vi "通过程序动态调整控件尺寸.vi"() -> ()   [LabVIEW 2010]
doc: "本VI是为《我和LabVIEW》一书编写的示例。\n关于本书的介绍请参考网页：\nhttp://ruanqizhen.spaces.live.com/blog/cns!5852D4F797C53FB6!4310.entry"
uses:
  C:/Program Files/National Instruments/LabVIEW 2010/resource/importtools/Common/Event/NISAST Event.lvclass
  <vilib>/Utility/miscctls.llb/LVPointTypeDef.ctl
panel:
  out "波形图":dbl[](graph)
  in  "停止":bool
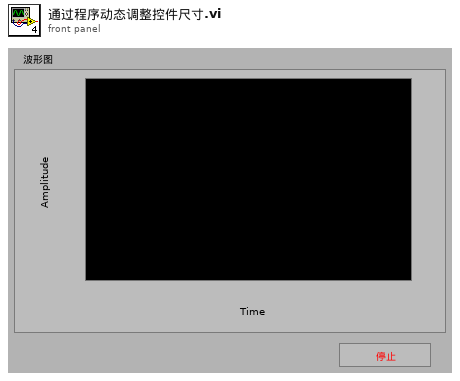
[diagram p1: front panel]
types:
  T1 = typedef "LVPointTypeDef.ctl" = cluster{"Horizontal":i16, "Vertical":i16}
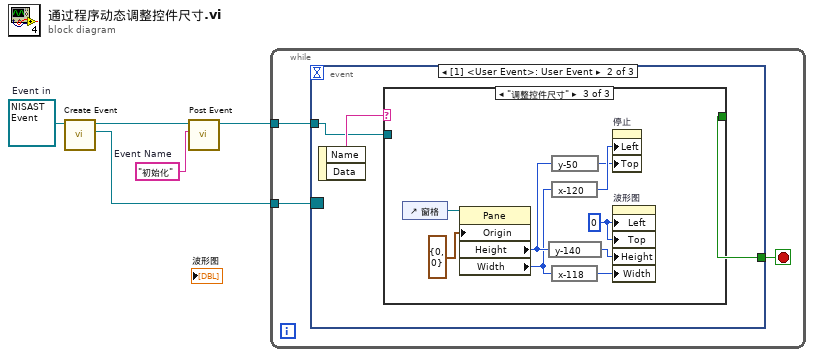
[diagram p0: block diagram]
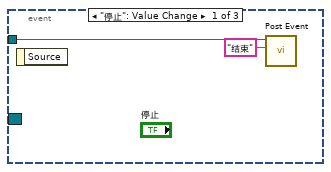
[diagram p2: hidden frame]
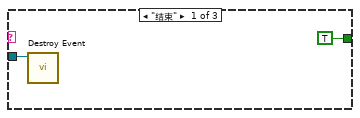
[diagram p3: hidden frame]
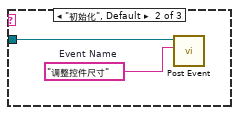
[diagram p4: hidden frame]
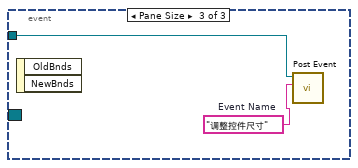
[diagram p5: hidden frame]
diagram:
  w1 = "初始化"  # Event Name
  w4 = refnum<class "NISAST Event.lvclass"> refnum  # Event in
  n1 = call-dynamic "Create Event.vi"("Event in"=w4) -> ("Event Registration Refnum"=w5:refnum<event-registration>, "Event out"=w3:refnum<class "NISAST Event.lvclass">)  [unwired: 1 in, 8 out]
  n2 = call-dynamic "Post Event.vi"("Event Name"=w1, "Event in"=w3) -> ("Event out"=w2:refnum<class "NISAST Event.lvclass">)  [unwired: 2 in, 7 out]
  n3 = while {
    tunnel: w5 -> [w8]
    tunnel: w2 -> [w6]
    stop <- w7 stop-if-true
    n4 = event shown="[1] <User Event>: User Event" {
      selector: w8 -> [_ _ _]
      dyn-events: _ -> [_ _ _]
      timeout: _ -> [_ _ _]
      tunnel: [_ w12 _] -> w7
      tunnel: w6 -> [w10 w11 w27]
      event "停止": Value Change {
        n5 = event-data() -> ()  [unwired: 2 out]
        n6 = call-dynamic "Post Event.vi"("Event Name"="结束", "Event in"=w10) -> ()  [unwired: 2 in, 8 out]
      }
      event User Event {
        n7 = event-data() -> ("Name"=w13:string)  [unwired: 2 out]
        n8 = case shown="\"调整控件尺寸\"" w13 {
          tunnel: [TRUE ("停止") _ _] -> w12
          tunnel: w11 -> [w14 w17 _]
          frame "结束" {
            n9 = call-dynamic "Destroy Event.vi"("Event in"=w14) -> ()  [unwired: 1 in, 10 out]
          }
          frame "初始化", Default {
            w16 = "调整控件尺寸"  # Event Name
            n10 = call-dynamic "Post Event.vi"("Event Name"=w16, "Event in"=w17) -> ()  [unwired: 2 in, 8 out]
          }
          frame "调整控件尺寸" {
            w22 = 0 ("Position:Left")
            n11 = control-ref of="窗格"() -> (w25:refnum<vi>)
            n12 = property class="Pane"(reference=w25, "Origin"=T1 {"Horizontal"=0, "Vertical"=0}) -> ("Height"=w21:u32, "Width"=w20:u32)  [unwired: 1 in, 2 out]
            n13 = expression code="y-140"(w21) -> (w24:u32)
            n14 = expression code="y-50"(w21) -> (w18:u32)
            n15 = expression code="x-120"(w20) -> (w19:u32)
            n16 = expression code="x-118"(w20) -> (w23:u32)
            n17 = property on="停止" class="Bool"("Left"=w19, "Top"=w18) -> ()  [unwired: 2 in, 2 out]
            n18 = property on="波形图" class="WFGraph (strict)"("Left"=w22, "Top"=w22, "Height"=w24, "Width"=w23) -> ()  [unwired: 2 in, 2 out]
          }
        }
      }
      event Pane Size {
        w28 = "调整控件尺寸"  # Event Name
        n19 = event-data() -> ()  [unwired: 3 out]
        n20 = call-dynamic "Post Event.vi"("Event Name"=w28, "Event in"=w27) -> ()  [unwired: 2 in, 8 out]
      }
    }
  }
